vi "File Transfer.vi"() -> ()   [LabVIEW 2017]
uses:
  <vilib>/FTP/NI_FTP.lvlib
panel:
  in  "local path":path
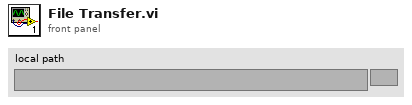
[diagram p1: front panel]
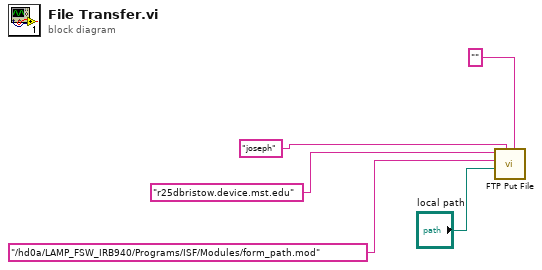
[diagram p0: block diagram]
diagram:
  n1 = call <vilib>:"FTP Put File.vi"("password"="", "user"="joseph", "local path"="local path", "remote path"="/hd0a/LAMP_FSW_IRB940/Programs/ISF/Modules/form_path.mod", "host"="r25dbristow.device.mst.edu") -> ()  [unwired: 5 in, 2 out]
